vi "Set Bias Voltage.vi"(8 "error in (no error)":errorcluster, 9 "Channel":i32, 10 "Bias Voltage (V)":dbl, 11 "Instrument.VoltageSource in":refnum<class "Instrument.VoltageSource.lvclass">) -> (0 "error out":errorcluster, 3 "Instrument.VoltageSource out":refnum<class "Instrument.VoltageSource.lvclass">)   [LabVIEW 2016, in "Instrument.VoltageSource.lvclass"]
uses:
  Instrument.VoltageSource.lvclass
  <userlib>/LevyLab/Levylab Instruments/Instrument Types/VSource/Instrument.VSource.lvclass
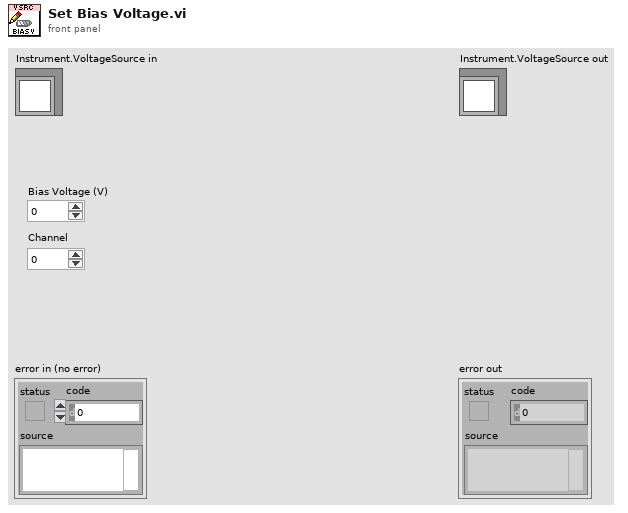
[diagram p1: front panel]
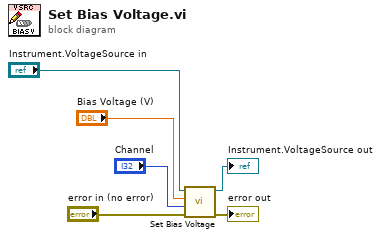
[diagram p0: block diagram]
diagram:
  n1 = call-parent "Set Bias Voltage.vi"("error in (no error)"="error in (no error)", "Channel"="Channel", "Bias Voltage (V)"="Bias Voltage (V)", "Instrument.VSource in"="Instrument.VoltageSource in") -> ("error out"=→"error out":errorcluster, "Instrument.VSource out"=→"Instrument.VoltageSource out":refnum<class "Instrument.VoltageSource.lvclass">)  [unwired: 6 in]
